vi "K7_Offset.vi"(7 "RF":T1 items=["RF_0", "RF_1", "RF_2", "RF_3"], 10 "Offset":u32[](array[numeric]) format="%x") -> (3 "Offset":u32)   [LabVIEW 2018]
uses:
  Types/RF.ctl
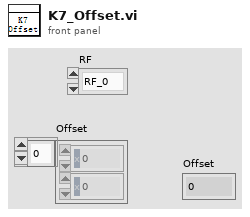
[diagram p1: front panel]
types:
  T1 = typedef "RF.ctl" = u16
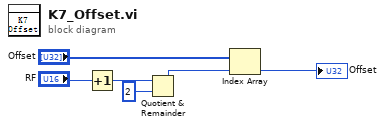
[diagram p0: block diagram]
diagram:
  n1 = Increment(x="RF") -> (x+1=w4:T1)
  n2 = Quotient & Remainder(x=w4, y=u16 2) -> (x-y*floor(x/y)=w2:T1)  [unwired: 1 out]
  n3 = Index Array(array="Offset", index=w2) -> (element=→"Offset":u32)
